vi "SavedSettingsReadFromINI.vi"(10 "Inifile path":path, 11 "SavedSettings in":refnum<vi>) -> ()   [LabVIEW 2021]
uses:
  <vilib>/Utility/config.llb/Read Key (I32).vi
  <vilib>/Utility/config.llb/Read Key (String).vi
  <vilib>/Utility/config.llb/NI_LVConfig.lvlib
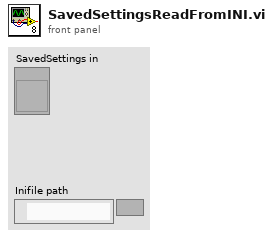
[diagram p1: front panel]
types:
  T1 = typedef "NI_LVConfig.lvlib/Config Data RefNum.ctl" = refnum<k1>
  T2 = cluster{"Indent Level":i32, "Title":string, "Date":string, "Description":string, "Values":string, "Apps":string, "VIs":string, "Opened":bool}
  T3 = cluster{"[0]":string, "[1]":string, "[2]":string, "[3]":string}
  T4 = cluster{"[0]":string, "[1]":string, "[2]":string}
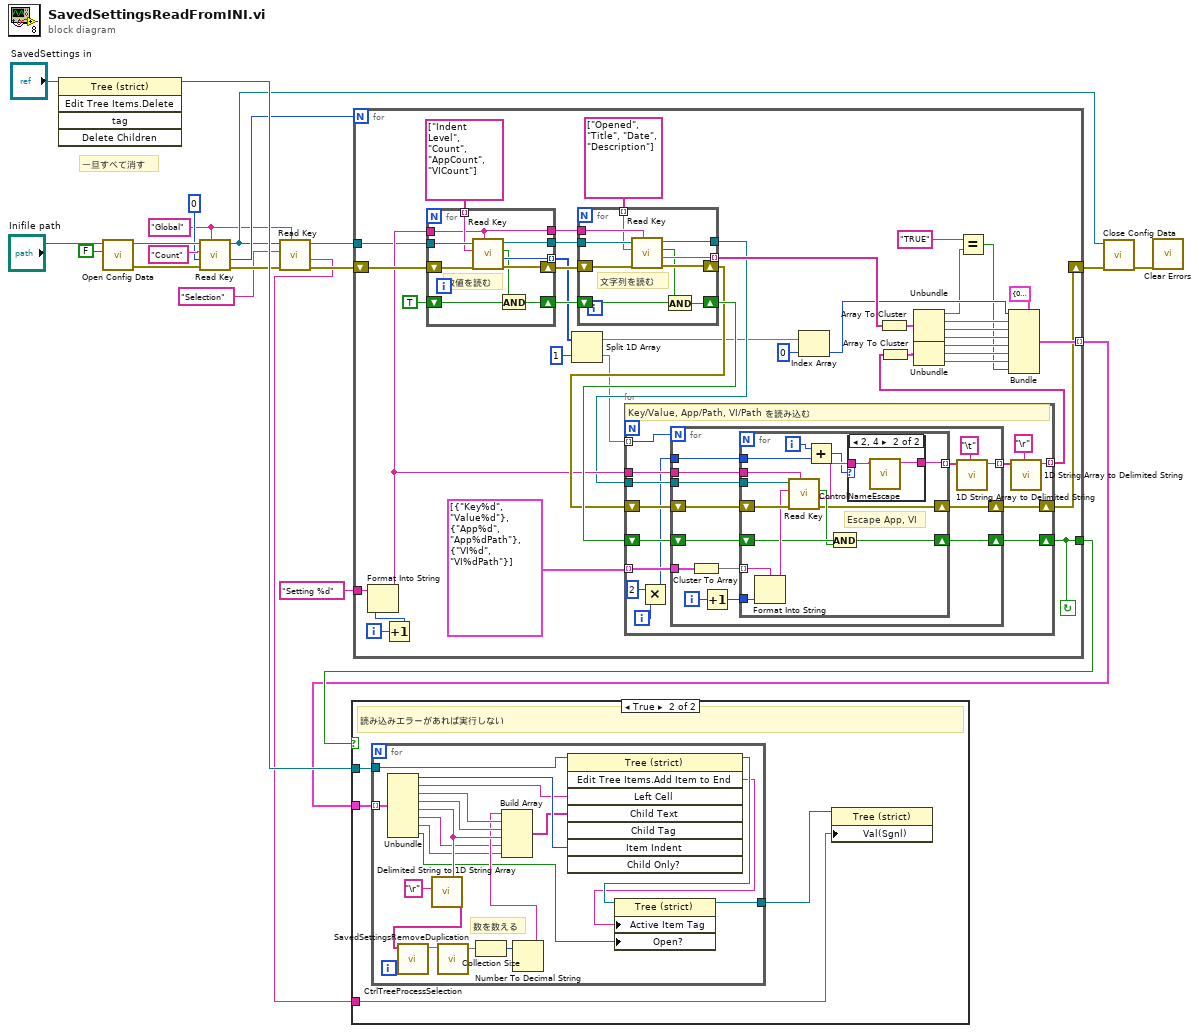
[diagram p0: block diagram]
diagram:
  w5 = "Global" ("section")
  # "一旦すべて消す"
  n1 = invoke class="Tree (strict)" method="Edit Tree Items.Delete"(reference="SavedSettings in") -> (reference out=w16:refnum<vi>)  [unwired: 4 in, 4 out]
  n2 = call <vilib>:"Open Config Data.vi"("create file if necessary (T)"=FALSE, "configuration file path"="Inifile path") -> ("error out"=w18:errorcluster, "refnum"=w20:T1)  [unwired: 7 in, 1 out]
  n3 = call-poly <vilib>:"Read Key.vi"("section"=w5, "error in (no error)"=w18, "default value"=0, "key"="Count", "refnum"=w20) -> ("error out"=w8:errorcluster, "value"=w14:i32, "refnum out"=w9:T1)  [unwired: 3 in, 1 out]
  n4 = call-poly <vilib>:"Read Key.vi"("section"=w5, "error in (no error)"=w8, "key"="Selection", "refnum"=w9) -> ("error out"=w6:errorcluster, "value"=w2:string, "refnum out"=w7:T1)  [unwired: 4 in, 1 out]
  n5 = for {
    N: w14 -> [_]
    tunnel: [w49] -> w12
    tunnel: [w47] -> w3 mode=indexing
    shift-right: [w41] -> w11
    shift-left: w6 -> [w59]
    tunnel: w7 -> [w34]
    tunnel: "Setting %d" ("format string") -> [w39]
    i -> [w60]
    stop <- w49 continue-if-true
    n6 = Increment(x=w60) -> (x+1=w61:i32)
    n7 = Format Into String(format string=w39, w61) -> (resulting string=w40:string)  [unwired: 2 in, 1 out]
    n8 = for {
      tunnel: w34 -> [w127]
      tunnel: w40 -> [w121]
      tunnel: string[] ["Indent Level", "Count", "AppCount", "VICount"] -> [w125] mode=indexing
      tunnel: [w124] -> w29 mode=indexing
      shift-right: [w123] -> w56
      shift-left: w59 -> [w126]
      tunnel: [w122] -> w58
      tunnel: [w121] -> w57
      shift-right: [w120] -> w52
      shift-left: TRUE ("found?") -> [w119]
      # "数値を読む"
      n9 = call-poly <vilib>:"Read Key.vi"("section"=w121, "error in (no error)"=w126, "key"=w125, "refnum"=w127) -> ("error out"=w123:errorcluster, "value"=w124:i32, "found?"=w118:bool, "refnum out"=w122:T1)  [unwired: 4 in]
      n10 = And(x=w118, y=w119) -> (x .and. y?=w120:bool)
    }
    n11 = Split 1D Array(array=w29, index=1) -> (first subarray=w28:i32[], second subarray=w30:i32[])
    n12 = for {
      tunnel: w58 -> [w117]
      tunnel: w57 -> [w115]
      tunnel: string[] ["Opened", "Title", "Date", "Description"] -> [w114] mode=indexing
      tunnel: [w113] -> w55 mode=indexing
      shift-right: [w112] -> w50
      shift-left: w56 -> [w116]
      tunnel: [w111] -> w35
      shift-right: [w110] -> w51
      shift-left: w52 -> [w109]
      # "文字列を読む"
      n13 = call-poly <vilib>:"Read Key.vi"("section"=w115, "error in (no error)"=w116, "key"=w114, "refnum"=w117) -> ("error out"=w112:errorcluster, "value"=w113:string, "found?"=w108:bool, "refnum out"=w111:T1)  [unwired: 4 in]
      n14 = And(x=w108, y=w109) -> (x .and. y?=w110:bool)
    }
    n15 = for {
      tunnel: w40 -> [w75]
      tunnel: w35 -> [w73]
      tunnel: [w70] -> w46 mode=indexing
      shift-right: [w66] -> w49
      shift-left: w51 -> [w67]
      tunnel: w30 -> [w69] mode=indexing
      tunnel: cluster{string, string}[] [{"Key%d", "Value%d"}, {"App%d", "App%dPath"}, {"VI%d", "VI%dPath"}] -> [w65] mode=indexing
      shift-right: [w68] -> w41
      shift-left: w50 -> [w74]
      i -> [w64]
      # "Key/Value, App/Path, VI/Path を読み込む"
      n16 = Multiply(x=2, y=w64) -> (x*y=w62:i32)
      n17 = for {
        N: w69 -> [_]
        shift-right: [w79] -> w68
        shift-left: w74 -> [w89]
        shift-right: [w80] -> w66
        shift-left: w67 -> [w87]
        tunnel: w75 -> [w84]
        tunnel: w73 -> [w86]
        tunnel: [w78] -> w72 mode=indexing
        tunnel: w65 -> [w77]
        tunnel: w62 -> [w76]
        i -> [w88]
        n18 = Cluster To Array(cluster=w77) -> (array=w83:string[])
        n19 = Increment(x=w88) -> (x+1=w85:i32)
        n20 = for {
          tunnel: w86 -> [w100]
          tunnel: w85 -> [w99]
          tunnel: w83 -> [w97] mode=indexing
          tunnel: w84 -> [w98]
          tunnel: [w93] -> w82 mode=indexing
          shift-right: [w96] -> w80
          shift-left: w87 -> [w102]
          shift-right: [w95] -> w79
          shift-left: w89 -> [w104]
          tunnel: w76 -> [w90]
          i -> [w92]
          # "Escape App, VI"
          n21 = Format Into String(format string=w97, w99) -> (resulting string=w103:string)  [unwired: 2 in, 1 out]
          n22 = call-poly <vilib>:"Read Key.vi"("section"=w98, "error in (no error)"=w104, "key"=w103, "refnum"=w100) -> ("error out"=w95:errorcluster, "value"=w94:string, "found?"=w101:bool)  [unwired: 4 in, 1 out]
          n23 = Add(x=w92, y=w90) -> (x+y=w91:i32)
          n24 = And(x=w102, y=w101) -> (x .and. y?=w96:bool)
          n25 = case shown="2, 4" w91 {
            tunnel: w94 -> [w105 w107]
            tunnel: [w105 w106] -> w93
            frame Default {
            }
            frame 2, 4 {
              n26 = call "ControlNameEscape.vi"("label"=w107) -> ("escaped string"=w106:string)  [unwired: 10 in]
            }
          }
        }
        n27 = call <vilib>:"1D String Array to Delimited String.vi"("delimiter"="\t", "string array"=w82) -> ("delimited string"=w78:string)  [unwired: 9 in]
      }
      n28 = call <vilib>:"1D String Array to Delimited String.vi"("delimiter"="\r", "string array"=w72) -> ("delimited string"=w70:string)  [unwired: 9 in]
    }
    n29 = Index Array(array=w28, index=0) -> (element=w32:i32)
    n30 = Array To Cluster(array=w55) -> (cluster=w54:T3)
    n31 = Array To Cluster(array=w46) -> (cluster=w45:T4)
    n32 = Unbundle(w54) -> ("[0]"=w23:string, "[1]"=w25:string, "[2]"=w26:string, "[3]"=w27:string)
    n33 = Unbundle(w45) -> ("[0]"=w44:string, "[1]"=w43:string, "[2]"=w42:string)
    n34 = Equal?(x="TRUE", y=w23) -> (x = y?=w22:bool)
    n35 = Bundle(cluster=T2 {"Indent Level"=0, "Title"="", "Date"="", "Description"="", "Values"="", "Apps"="", "VIs"="", "Opened"=TRUE}, "Indent Level"=w32, "Title"=w25, "Date"=w26, "Description"=w27, "Values"=w44, "Apps"=w43, "VIs"=w42, "Opened"=w22) -> (w47:T2)
  }
  n36 = case shown="True" w12 {
    tunnel: w3 -> [_ w131]
    tunnel: w16 -> [_ w130]
    tunnel: w2 -> [_ w128]
    frame False {
    }
    frame True {
      # "読み込みエラーがあれば実行しない"
      n37 = for {
        tunnel: w131 -> [w151] mode=indexing
        tunnel: w130 -> [w136]
        tunnel: [w132] -> w129
        # "数を数える"
        n38 = Unbundle(w151) -> ("Indent Level"=w150:i32, "Title"=w149:string, "Date"=w140:string, "Description"=w147:string, "Values"=w143:string, "Apps"=w138:string, "VIs"=w137:string, "Opened"=w133:bool)
        n39 = call <vilib>:"Delimited String to 1D String Array.vi"("delimiter"="\r", "delimited string"=w143) -> ("string array"=w141:string[])  [unwired: 9 in]
        n40 = call "CtrlTreeProcessSelection.vi"("Selection"=w141) -> ("Map"=w144:map{string, string})  [unwired: 10 in]
        n41 = call "SavedSettingsRemoveDuplication.vi"("Saved Values"=w144) -> ("Saved Values (children removed)"=w146:map{string, string})  [unwired: 9 in, 1 out]
        n42 = Collection Size(1:w146) -> (0:w145:i32)
        n43 = Number To Decimal String(number=w145) -> (decimal integer string=w139:string)  [unwired: 1 in]
        n44 = Build Array(w139, w140, w147, w143, w138, w137) -> (w148:string[])
        n45 = invoke class="Tree (strict)" method="Edit Tree Items.Add Item to End"(reference=w136, "Left Cell"=w149, "Child Text"=w148, "Item Indent"=w150) -> (reference out=w135:refnum<vi>, "Edit Tree Items:Add Item to End"=w134:string)  [unwired: 4 in, 6 out]
        n46 = property class="Tree (strict)"(reference=w135, "Active Item Tag"=w134, "Open?"=w133) -> (reference out=w132:refnum<vi>)  [unwired: 1 in, 1 out]
      }
      n47 = property class="Tree (strict)"(reference=w129, "Val(Sgnl)"=w128) -> ()  [unwired: 1 in, 2 out]
    }
  }
  n48 = call <vilib>:"Close Config Data.vi"("error in (no error)"=w11, "refnum"=w9) -> ("error out"=w1:errorcluster)  [unwired: 8 in, 1 out]
  n49 = call <vilib>:"Clear Errors.vi"("error in (no error)"=w1) -> ()  [unwired: 5 in, 2 out]
